vi "TrapProfile_TimeLeftUntil.vi"(9 "TargetDistance":dbl, 11 "TRAPEZOID_PROFILE":T1 {"Goal"."Velocity" format="%16_6e"; "Goal"."Position" format="%16_6e"; "Initial"."Velocity" format="%16_6e"; "Initial"."Position" format="%16_6e"; "Constraints"."MaxAcceleration" format="%16_6e"; "Constraints"."MaxVelocity" format="%16_6e"; "EndDecel" format="%16_6e"; "EndFullSpeed" format="%16_6e"; "EndAccel" format="%16_6e"}) -> (3 "TimeLeft":dbl)   [LabVIEW 2019, in "Trajectory_Library.lvlib"]
doc: "Returns the time left until a target distance in the profile is reached.\n \nInputs:\n - Trapezoid_Profile -- The Trapezoid_Profile data cluster\n - target -- The target distance.\n\nOutputs:\n - timeLeft -- Time remaining to reach target (seconds)"
uses:
  Trajectory_Library.lvlib
  TRAPEZOID_PROFILE.ctl
  TRAPEZOID_PROFILE_CONSTRAINT.ctl
  TRAPEZOID_PROFILE_STATE.ctl
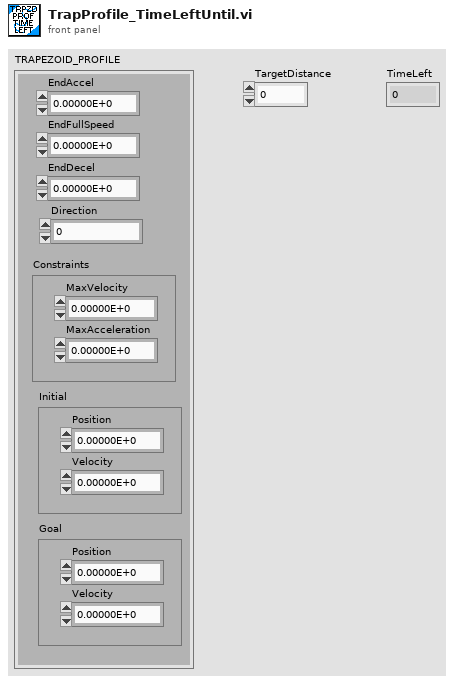
[diagram p1: front panel]
types:
  T1 = typedef "Trajectory_Library.lvlib/TRAPEZOID_PROFILE.ctl" = cluster{"EndAccel":dbl, "EndFullSpeed":dbl, "EndDecel":dbl, "Direction":i32, "Constraints":T2, "Initial":T3, "Goal":T3}
  T2 = typedef "Trajectory_Library.lvlib/TRAPEZOID_PROFILE_CONSTRAINT.ctl" = cluster{"MaxVelocity":dbl, "MaxAcceleration":dbl}
  T3 = typedef "Trajectory_Library.lvlib/TRAPEZOID_PROFILE_STATE.ctl" = cluster{"Position":dbl, "Velocity":dbl}
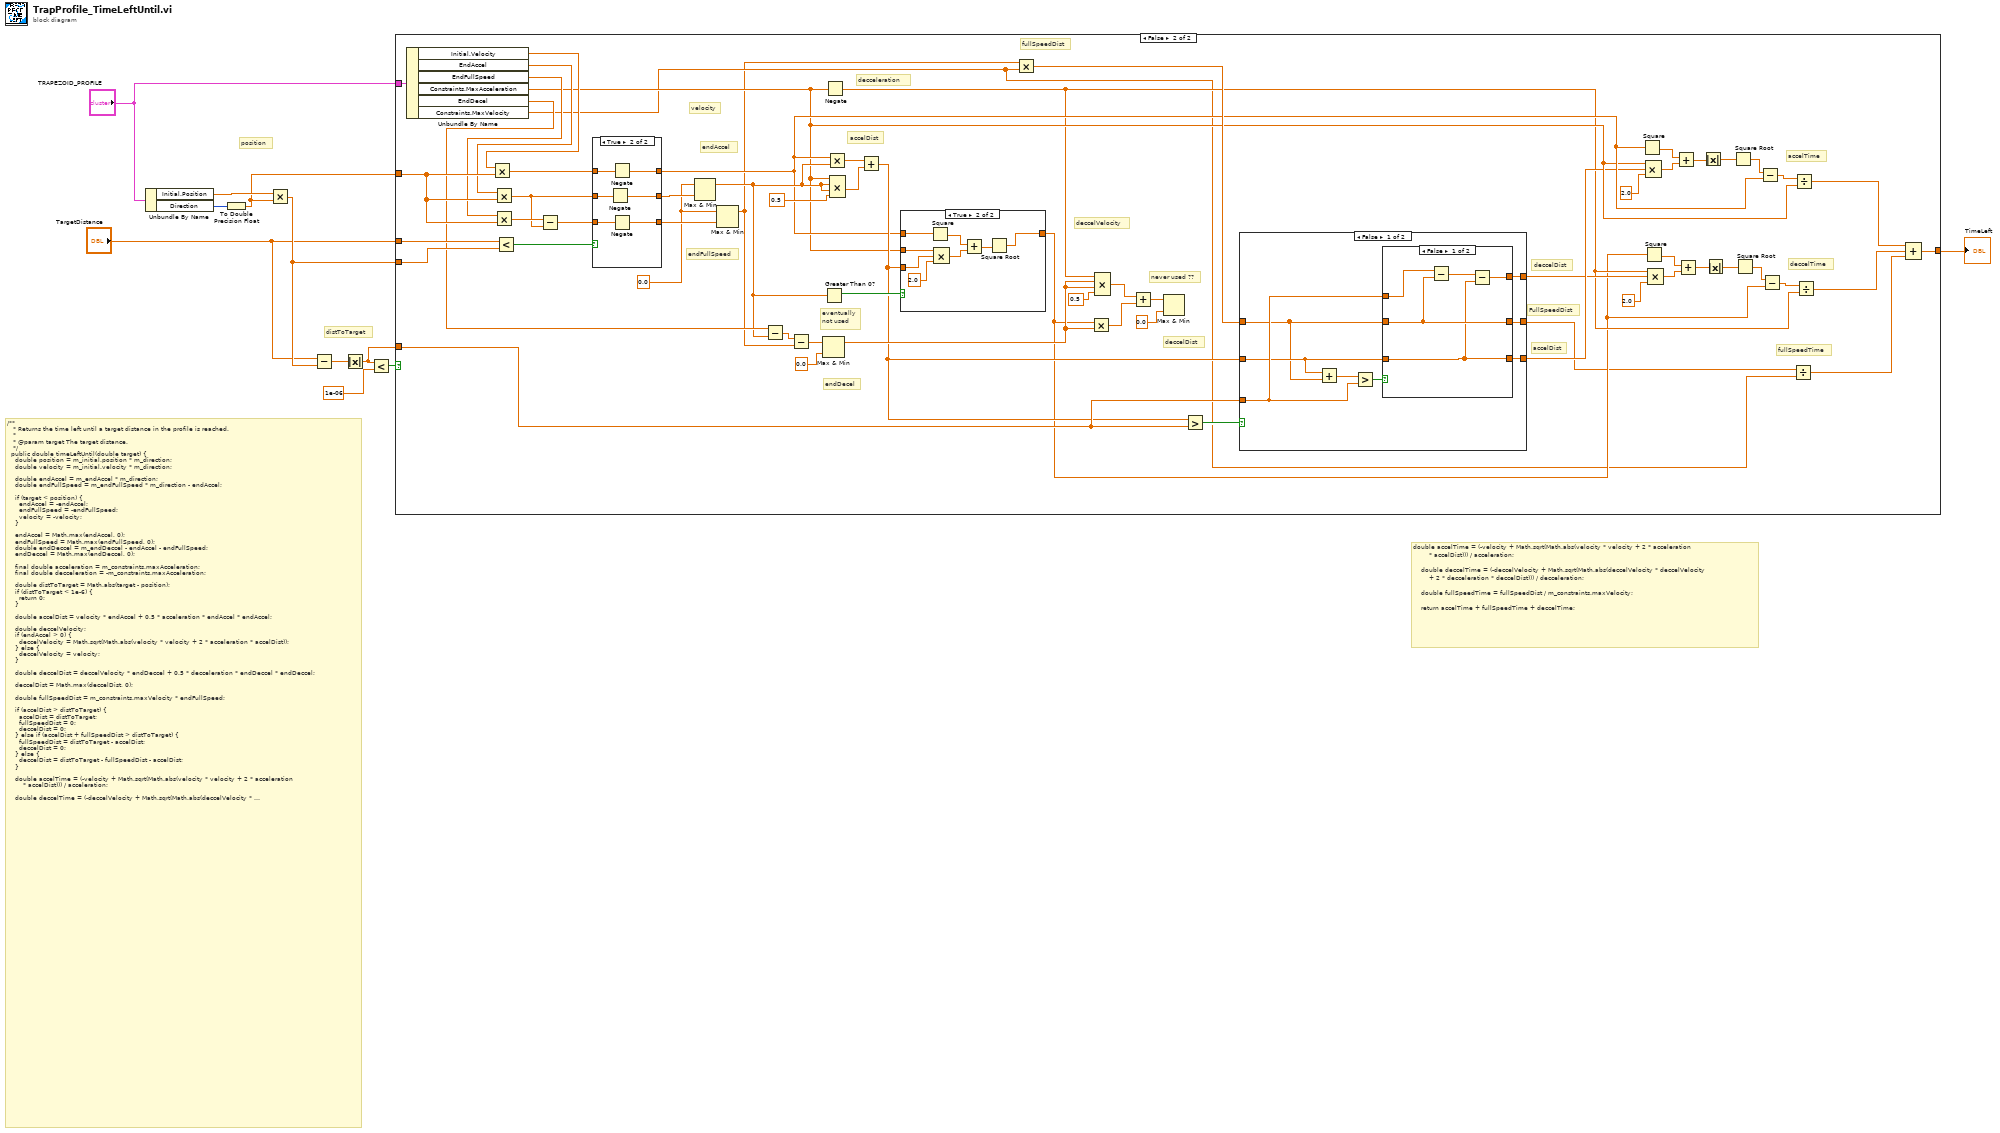
[diagram p0: block diagram]
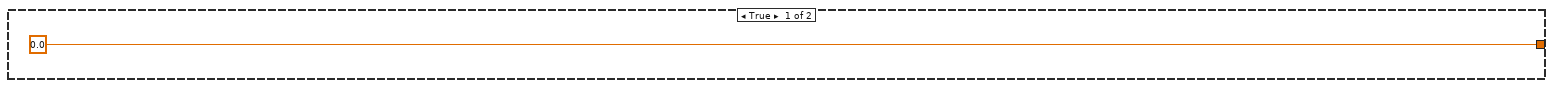
[diagram p2: hidden frame]
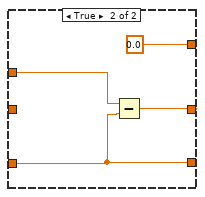
[diagram p3: hidden frame]
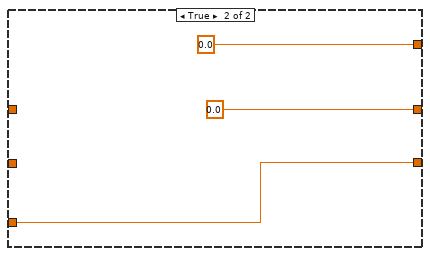
[diagram p4: hidden frame]
diagram:
  # "double accelTime = (-velocity + Math.sqrt(Math.abs(velocity * velocity + 2 * acceleration\n        * accelDist))) / acceleration;\n\n    double deccelTime = (-deccelVelocity + Math.sqrt(Math.abs(deccelVelocity * deccelVelocity\n        + 2 * decceleration * deccelDist))) / decceleration;\n\n    double fullSpeedTime = fullSpeedDist / m_constraints.maxVelocity;\n\n    return accelTime + fullSpeedTime + deccelTime;"
  # "distToTarget"
  # "position"
  # "/**\n   * Returns the time left until a target distance in the profile is reached.\n   *\n   * @param target The target distance.\n   */\n  public double timeLeftUntil(double target) {\n    double position = m_initial.position * m_direction;\n    double velocity = m_initial.velocity * m_direction;\n\n    double endAccel = m_endAccel * m_direction;\n    double endFullSpeed = m_endFullSpeed * m_direction - endAccel;\n\n    if (target < position) {\n      endAccel = -endAccel;\n      endFullSpeed = -endFullSpeed;\n      velocity = -velocity;\n    }\n\n    endAccel = Math.max(endAccel, 0);\n    endFullSpeed = Math.max(endFullSpeed, 0);\n    double endDeccel = m_endDeccel - endAccel - endFullSpeed;\n    endDeccel = Math.max(endDeccel, 0);\n\n    final double acceleration = m_constraints.maxAcceleration;\n    final double decceleration = -m_constraints.maxAcceleration;\n\n    double distToTarget = Math.abs(target - position);\n    if (distToTarget < 1e-6) {\n      return 0;\n    }\n\n    double accelDist = velocity * endAccel + 0.5 * acceleration * endAccel * endAccel;\n\n    double deccelVelocity;\n    if (endAccel > 0) {\n      deccelVelocity = Math.sqrt(Math.abs(velocity * velocity + 2 * acceleration * accelDist));\n    } else {\n      deccelVelocity = velocity;\n    }\n\n    double deccelDist = deccelVelocity * endDeccel + 0.5 * decceleration * endDeccel * endDeccel;\n\n    deccelDist = Math.max(deccelDist, 0);\n\n    double fullSpeedDist = m_constraints.maxVelocity * endFullSpeed;\n\n    if (accelDist > distToTarget) {\n      accelDist = distToTarget;\n      fullSpeedDist = 0;\n      deccelDist = 0;\n    } else if (accelDist + fullSpeedDist > distToTarget) {\n      fullSpeedDist = distToTarget - accelDist;\n      deccelDist = 0;\n    } else {\n      deccelDist = distToTarget - fullSpeedDist - accelDist;\n    }\n\n    double accelTime = (-velocity + Math.sqrt(Math.abs(velocity * velocity + 2 * acceleration\n        * accelDist))) / acceleration;\n\n    double deccelTime = (-deccelVelocity + Math.sqrt(Math.abs(deccelVelocity * deccelVelocity\n        + 2 * decceleration * deccelDist))) / decceleration;\n\n    double fullSpeedTime = fullSpeedDist / m_constraints.maxVelocity;\n\n    return accelTime + fullSpeedTime + deccelTime;\n  }"
  n1 = Unbundle By Name("TRAPEZOID_PROFILE") -> ("Initial.Position"=w10:dbl, "Direction"=w11:i32)
  n2 = To Double Precision Float(number=w11) -> (double precision float=w4:dbl)
  n3 = Multiply(x=w10, y=w4) -> (x*y=w6:dbl)
  n4 = Subtract(x="TargetDistance", y=w6) -> (x-y=w9:dbl)
  n5 = Absolute Value(x=w9) -> (abs(x)=w1:dbl)
  n6 = Less?(x=w1, y=1e-06) -> (x < y?=w7:bool)
  n7 = case shown="False" w7 {
    tunnel: w6 -> [_ w66]
    tunnel: "TargetDistance" -> [_ w65]
    tunnel: w4 -> [_ w58]
    tunnel: "TRAPEZOID_PROFILE" -> [_ w60]
    tunnel: [0.0 w14] -> w2
    tunnel: w1 -> [_ w42]
    frame True {
    }
    frame False {
      w71 = 0.0
      # "decceleration"
      # "eventually\nnot used"
      # "fullSpeedTime"
      # "never used ??"
      # "deccelTime"
      # "accelTime"
      # "deccelDist"
      # "FullSpeedDist"
      # "accelDist"
      # "fullSpeedDist"
      # "deccelDist"
      # "deccelVelocity"
      # "accelDist"
      # "endDecel"
      # "endFullSpeed"
      # "endAccel"
      # "velocity"
      n8 = Unbundle By Name(w60) -> ("Initial.Velocity"=w59:dbl, "EndAccel"=w57:dbl, "EndFullSpeed"=w44:dbl, "Constraints.MaxAcceleration"=w31:dbl, "EndDecel"=w56:dbl, "Constraints.MaxVelocity"=w18:dbl)
      n9 = Multiply(x=w59, y=w58) -> (x*y=w61:dbl)
      n10 = Multiply(x=w57, y=w58) -> (x*y=w62:dbl)
      n11 = Multiply(x=w44, y=w58) -> (x*y=w67:dbl)
      n12 = Less?(x=w65, y=w66) -> (x < y?=w64:bool)
      n13 = Subtract(x=w67, y=w62) -> (x-y=w63:dbl)
      n14 = case shown="True" w64 {
        tunnel: w63 -> [w103 w111]
        tunnel: w62 -> [w104 w110]
        tunnel: w61 -> [w105 w109]
        tunnel: [w105 w108] -> w33
        tunnel: [w104 w107] -> w73
        tunnel: [w103 w106] -> w72
        frame False {
        }
        frame True {
          n15 = Negate(x=w110) -> (-x=w107:dbl)
          n16 = Negate(x=w109) -> (-x=w108:dbl)
          n17 = Negate(x=w111) -> (-x=w106:dbl)
        }
      }
      n18 = Max & Min(x=w71, y=w73) -> (max(x,y)=w51:dbl)  [unwired: 1 out]
      n19 = Max & Min(x=w71, y=w72) -> (max(x,y)=w13:dbl)  [unwired: 1 out]
      n20 = Subtract(x=w56, y=w51) -> (x-y=w70:dbl)
      n21 = Subtract(x=w70, y=w13) -> (x-y=w69:dbl)
      n22 = Max & Min(x=w69, y=0.0) -> (max(x,y)=w50:dbl)  [unwired: 1 out]
      n23 = Greater Than 0?(x=w51) -> (x > 0?=w52:bool)
      n24 = Negate(x=w31) -> (-x=w21:dbl)
      n25 = Multiply(x=w33, y=w51) -> (x*y=w54:dbl)
      n26 = Compound Arithmetic op=MULTIPLY(w31, w51, w51, 0.5 ("value")) -> (w53:dbl)
      n27 = Add(x=w54, y=w53) -> (x+y=w40:dbl)
      n28 = case shown="True" w52 {
        tunnel: w33 -> [w94 w102]
        tunnel: [w94 w95] -> w20
        tunnel: w31 -> [_ w101]
        tunnel: w40 -> [_ w100]
        frame False {
        }
        frame True {
          n29 = Square(x=w102) -> (x^2=w98:dbl)
          n30 = Compound Arithmetic op=MULTIPLY(w101, w100, 2.0 ("value")) -> (w97:dbl)
          n31 = Add(x=w98, y=w97) -> (x+y=w96:dbl)
          n32 = Square Root(x=w96) -> (sqrt(x)=w95:dbl)
        }
      }
      n33 = Multiply(x=w13, y=w18) -> (x*y=w41:dbl)
      n34 = Multiply(x=w20, y=w50) -> (x*y=w47:dbl)
      n35 = Compound Arithmetic op=MULTIPLY(w21, w50, w50, 0.5 ("value")) -> (w48:dbl)
      n36 = Add(x=w48, y=w47) -> (x+y=w45:dbl)
      n37 = Max & Min(x=w45, y=0.0) -> ()  [unwired: 2 out]
      n38 = Greater?(x=w40, y=w42) -> (0:w43:bool)
      n39 = case shown="False" w43 {
        tunnel: w42 -> [w77 w93]
        tunnel: [w80 w93] -> w23
        tunnel: [w81 0.0] -> w19
        tunnel: [w79 0.0] -> w22
        tunnel: w41 -> [w74 _]
        tunnel: w40 -> [w75 _]
        frame False {
          n40 = Add(x=w75, y=w74) -> (x+y=w76:dbl)
          n41 = Greater?(x=w76, y=w77) -> (0:w78:bool)
          n42 = case shown="False" w78 {
            tunnel: [w85 w89] -> w81
            tunnel: w74 -> [w85 _]
            tunnel: w75 -> [w83 w87]
            tunnel: [w83 w87] -> w80
            tunnel: [w82 0.0] -> w79
            tunnel: w77 -> [w86 w88]
            frame False {
              n43 = Subtract(x=w86, y=w85) -> (x-y=w84:dbl)
              n44 = Subtract(x=w84, y=w83) -> (x-y=w82:dbl)
            }
            frame True {
              n45 = Subtract(x=w88, y=w87) -> (x-y=w89:dbl)
            }
          }
        }
        frame True {
        }
      }
      n46 = Square(x=w33) -> (x^2=w38:dbl)
      n47 = Square(x=w20) -> (x^2=w29:dbl)
      n48 = Compound Arithmetic op=MULTIPLY(w31, w23, 2.0 ("value")) -> (w37:dbl)
      n49 = Compound Arithmetic op=MULTIPLY(w21, w22, 2.0 ("value")) -> (w28:dbl)
      n50 = Add(x=w38, y=w37) -> (x+y=w36:dbl)
      n51 = Add(x=w29, y=w28) -> (x+y=w27:dbl)
      n52 = Absolute Value(x=w36) -> (abs(x)=w35:dbl)
      n53 = Absolute Value(x=w27) -> (abs(x)=w26:dbl)
      n54 = Square Root(x=w35) -> (sqrt(x)=w34:dbl)
      n55 = Square Root(x=w26) -> (sqrt(x)=w25:dbl)
      n56 = Subtract(x=w34, y=w33) -> (x-y=w32:dbl)
      n57 = Subtract(x=w25, y=w20) -> (x-y=w24:dbl)
      n58 = Divide(x=w19, y=w18) -> (x/y=w15:dbl)
      n59 = Divide(x=w32, y=w31) -> (x/y=w17:dbl)
      n60 = Divide(x=w24, y=w21) -> (x/y=w16:dbl)
      n61 = Compound Arithmetic op=ADD(w17, w16, w15) -> (w14:dbl)
    }
  }
  "TimeLeft" <- w2
